vi "RPM2FF.vi"(11 "RPM":dbl=1550.0 format="%#_13g") -> (3 "FF value":dbl)   [LabVIEW 2016]
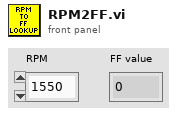
[diagram p1: front panel]
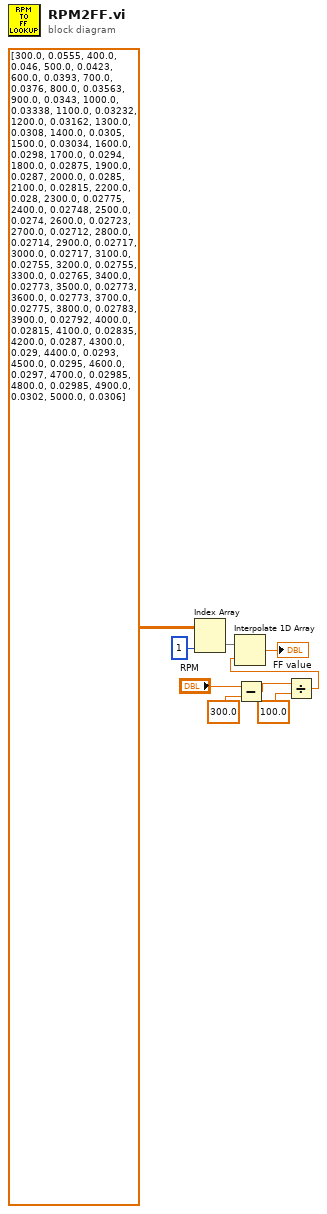
[diagram p0: block diagram]
diagram:
  n1 = Index Array(array=dbl[][] [[300.0, 0.0555], [400.0, 0.046], [500.0, 0.0423], [600.0, 0.0393], [700.0, 0.0376], [800.0, 0.03563], [900.0, 0.0343], [1000.0, 0.03338], [1100.0, 0.03232], [1200.0, 0.03162], [1300.0, 0.0308], [1400.0, 0.0305], [1500.0, 0.03034], [1600.0, 0.0298], [1700.0, 0.0294], [1800.0, 0.02875], [1900.0, 0.0287], [2000.0, 0.0285], [2100.0, 0.02815], [2200.0, 0.028], [2300.0, 0.02775], [2400.0, 0.02748], [2500.0, 0.0274], [2600.0, 0.02723], [2700.0, 0.02712], [2800.0, 0.02714], [2900.0, 0.02717], [3000.0, 0.02717], [3100.0, 0.02755], [3200.0, 0.02755], [3300.0, 0.02765], [3400.0, 0.02773], [3500.0, 0.02773], [3600.0, 0.02773], [3700.0, 0.02775], [3800.0, 0.02783], [3900.0, 0.02792], [4000.0, 0.02815], [4100.0, 0.02835], [4200.0, 0.0287], [4300.0, 0.029], [4400.0, 0.0293], [4500.0, 0.0295], [4600.0, 0.0297], [4700.0, 0.02985], [4800.0, 0.02985], [4900.0, 0.0302], [5000.0, 0.0306]], index (col)=1 ("disabled index (col)")) -> (element=w3:dbl[])  [unwired: 1 in]
  n2 = Subtract(x="RPM", y=300.0) -> (x-y=w8:dbl)
  n3 = Divide(x=w8, y=100.0) -> (x/y=w9:dbl)
  n4 = Interpolate 1D Array(1:w9, 2:w3) -> (0:→"FF value":dbl)
